vi "vi server BAE6.1.vi"(0 "VI ref in":refnum<vi>, 11 "error in":errorcluster) -> (4 "VI ref out":refnum<vi>, 10 "FP.WinBounds":T1, 15 "error out":errorcluster)   [LabVIEW 2014]
doc: "VI Server\n\nSets the vi front panel to its starting posiition, which is in the center of the monitor.\n\nBeverly Abadinnes\nPHY 350\nE6"
uses:
  <vilib>/Utility/miscctls.llb/LVRectTypeDef.ctl
panel:
  # "VI Server BAE6"
  # "Beverly Abadines\nPhys 350\nE6"
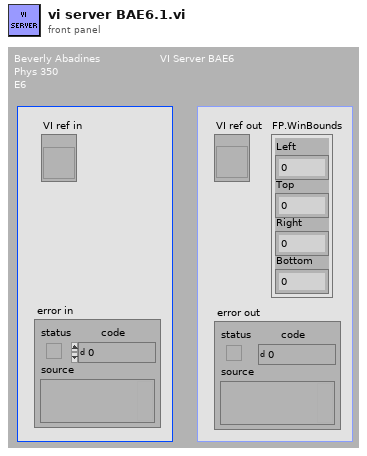
[diagram p1: front panel]
types:
  T1 = typedef "LVRectTypeDef.ctl" = cluster{"Left":i16, "Top":i16, "Right":i16, "Bottom":i16}
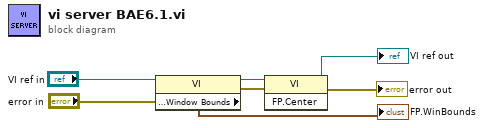
[diagram p0: block diagram]
diagram:
  n1 = property class="VI"(reference="VI ref in", error in="error in") -> (reference out=w7:refnum<vi>, error out=w6:errorcluster, "Front Panel Window:Window Bounds"=→"FP.WinBounds":T1)
  n2 = invoke class="VI" method="FP.Center"(reference=w7, error in=w6) -> (reference out=→"VI ref out":refnum<vi>, error out=→"error out":errorcluster)  [unwired: 1 in, 1 out]
